vi "CopyPixmapToImageIgnoreMaskGreyscale.vi"(8 "error in (no error)":errorcluster, 10 "Greyscale Image Destination":refnum<data-value>, 11 "Pixmap Image Data":T1) -> (0 "error out":errorcluster, 3 "Greyscale Image Destination (duplicate)":refnum<data-value>)   [LabVIEW 2020, in "g_ar_toolkit.image.lvlib"]
uses:
  g_ar_toolkit.image.lvlib
  <vilib>/picture/picture.llb/imagedata.ctl
  FixPixmapColourArraySize.vi
  Default8bitColourMap.vi
  <vilib>/Utility/error.llb/Error Cluster From Error Code.vi
  80b1166a-8c06-443b-b271-eb6a715622f7.vi
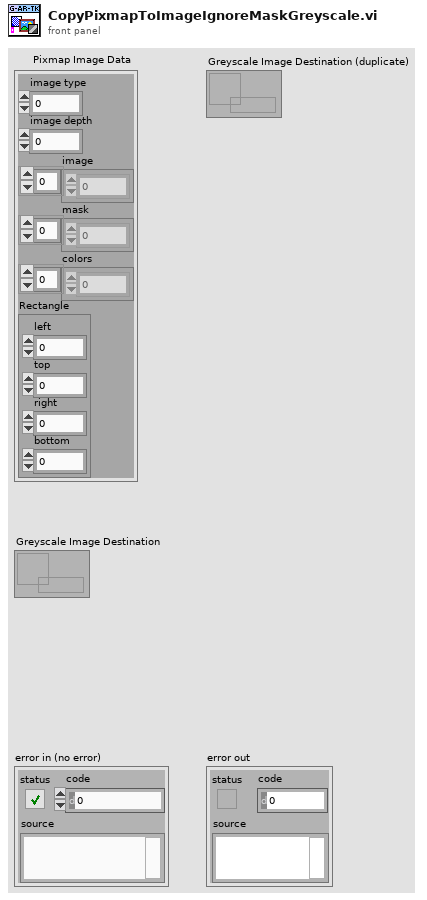
[diagram p1: front panel]
types:
  T1 = typedef "imagedata.ctl" = cluster{"image type":i32, "image depth":i32, "image":u8[], "mask":u8[], "colors":u32[], "Rectangle":cluster{"left":i16, "top":i16, "right":i16, "bottom":i16}}
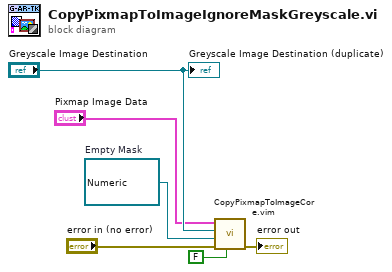
[diagram p0: block diagram]
diagram:
  w1 = refnum<data-value> refnum  # Empty Mask
  n1 = call "CopyPixmapToImageCore.vim"("Has Mask"=FALSE, "error in (no error)"="error in (no error)", "Mask Image"=w1, "Destination Image"="Greyscale Image Destination", "image data"="Pixmap Image Data") -> ("error out"=→"error out":errorcluster)  [unwired: 6 in]
  "Greyscale Image Destination (duplicate)" <- "Greyscale Image Destination"
